vi "DETECT REFERENCE LINE.vi"   [LabVIEW 2016, in "Test2.lvrbt"]
uses:
  Test2.lvrbt
  <vilib>/NXT/Subs/ColorSensorColors.ctl
  <vilib>/NXT/Block Support/NXT_InputPort.ctl
  <vilib>/NXT/Hardware/Plugins/Tetrix DC Motor/TetrixDCMotorAddress.ctl
  <vilib>/NXT/NXTIO Xnodes/NXTIONodeSubVIs/TETRIX IO Move DC Motors.vi
  <vilib>/NXT/Dual Mode Library/Waits/Wait_Num.vi
  <vilib>/NXT/NXTIO Xnodes/NXTIONodeSubVIs/TETRIX IO Stop DC Motors.vi
  <vilib>/NXT/Dual Mode Library/Waits/Wait_EV3_Color_Color.vi
  <vilib>/NXT/Subs/LVHSConnector.ctl
  <vilib>/NXT/NXTIO Xnodes/AddressXNode/NXTIOAddress.xnode
  <vilib>/NXT/NXTIO Xnodes/NXTIOXNode/NXTIO.xnode
  <vilib>/NXT/LegoClasses/BrickReference/BrickReference.lvclass
types:
  T1 = typedef "NXT_InputPort.ctl" = u32
  T2 = typedef "ColorSensorColors.ctl" = enum16{"No Color", "Black", "Blue", "Green", "Yellow", "Red", "White", "Brown"}
  T3 = typedef "TetrixDCMotorAddress.ctl" = i32
  T4 = typedef "LVHSConnector.ctl" = refnum<class "BrickReference.lvclass">
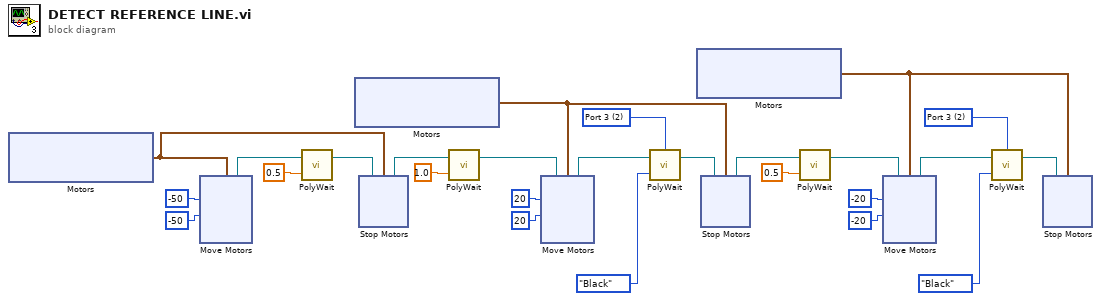
[diagram p0: block diagram]
diagram:
  w2 = T1 2 items=["Port 1", "Port 2", "Port 3", "Port 4"] ("Port (Port 1)")
  w11 = T1 2 items=["Port 1", "Port 2", "Port 3", "Port 4"] ("Port (Port 1)")
  n1 = xnode "Motors"() -> ("Motor"=w21:cluster{"TetrixDCMotor":T3, "TetrixDCMotor":T3})
  n2 = xnode "Move Motors"("Power/Speed 2"=i8 -50, "Power/Speed 1"=i8 -50, "Motors"=w21) -> ("NXT/EV3"=w24:T4)  [unwired: 1 in]
  n3 = call-poly <vilib>:"PolyWait.vi"("Time (1 sec)"=sgl 0.5, "NXT/EV3"=w24) -> ("NXT/EV3"=w23:T4)  [unwired: 2 in]
  n4 = xnode "Motors"() -> ("Motor"=w16:cluster{"TetrixDCMotor":T3, "TetrixDCMotor":T3})
  n5 = xnode "Stop Motors"("Motors"=w21, "NXT/EV3"=w23) -> ("NXT/EV3"=w14:T4)
  n6 = call-poly <vilib>:"PolyWait.vi"("Time (1 sec)"=sgl 1.0, "NXT/EV3"=w14) -> ("NXT/EV3"=w13:T4)  [unwired: 2 in]
  n7 = xnode "Move Motors"("Power/Speed 2"=i8 20, "Power/Speed 1"=i8 20, "Motors"=w16, "NXT/EV3"=w13) -> ("NXT/EV3"=w18:T4)
  n8 = call-poly <vilib>:"PolyWait.vi"("Color (Red)"=ColorSensorColors."Black", "NXT/EV3"=w18, "Port (Port 1)"=w11) -> ("NXT/EV3"=w17:T4)  [unwired: 1 in]
  n9 = xnode "Motors"() -> ("Motor"=w6:cluster{"TetrixDCMotor":T3, "TetrixDCMotor":T3})
  n10 = xnode "Stop Motors"("Motors"=w16, "NXT/EV3"=w17) -> ("NXT/EV3"=w1:T4)
  n11 = call-poly <vilib>:"PolyWait.vi"("Time (1 sec)"=sgl 0.5, "NXT/EV3"=w1) -> ("NXT/EV3"=w4:T4)  [unwired: 2 in]
  n12 = xnode "Move Motors"("Power/Speed 2"=i8 -20, "Power/Speed 1"=i8 -20, "Motors"=w6, "NXT/EV3"=w4) -> ("NXT/EV3"=w8:T4)
  n13 = call-poly <vilib>:"PolyWait.vi"("Color (Red)"=ColorSensorColors."Black", "NXT/EV3"=w8, "Port (Port 1)"=w2) -> ("NXT/EV3"=w7:T4)  [unwired: 1 in]
  n14 = xnode "Stop Motors"("Motors"=w6, "NXT/EV3"=w7) -> ()  [unwired: 1 out]
